vi "acq_eeg_read.vi"(7 "Marker Queue":refnum<queue>, 8 "error in (no error)":errorcluster, 10 "variant in":variant, 11 "eeg_device":T1) -> (0 "error out":errorcluster, 1 "Next Acq State":string, 2 "Variant out":variant, 3 "eeg samples":dbl[][](array[numeric]), 5 "Marker Queue Out":refnum<queue>)   [LabVIEW 2013]
uses:
  <vilib>/NIOSC/Address Space Node.ctl
  gui/type_def/device.ctl
  <vilib>/NI/Emotiv Toolkit/Emotiv Task.lvclass
  <vilib>/NI/Emotiv Toolkit/Utilities/EE DataChannels_enum.ctl
  <vilib>/OpenBCI/Comm Protocol/Control Def/openbci_device.ctl
  <vilib>/OpenBCI/Comm Protocol/Control Def/channel_count.ctl
  gui/type_def/file_stream.ctl
  <vilib>/NIOSC/Argument to Float32 Data.vi
  <vilib>/NIOSC/Generate Error.vi
  <vilib>/NIOSC/NI_OSC.lvlib
  <vilib>/NI/LabVIEW - NeuroSky Driver/NeuroSky Driver.lvlib
  <vilib>/NI/LabVIEW - NeuroSky Driver/NeuroSky Driver/ThinkGear Read/ThinkGear MultiSample Read Raw.vi
panel:
  out "Livesign Msg":bool
  out "ECG Chart":u32[](graph)
  out "Acc Chart":dbl[][](graph)
  out "Respiration Chart":u32[](graph)
  in  "NeuroSky Task Out":T2
  in  "muse cluster out":T4
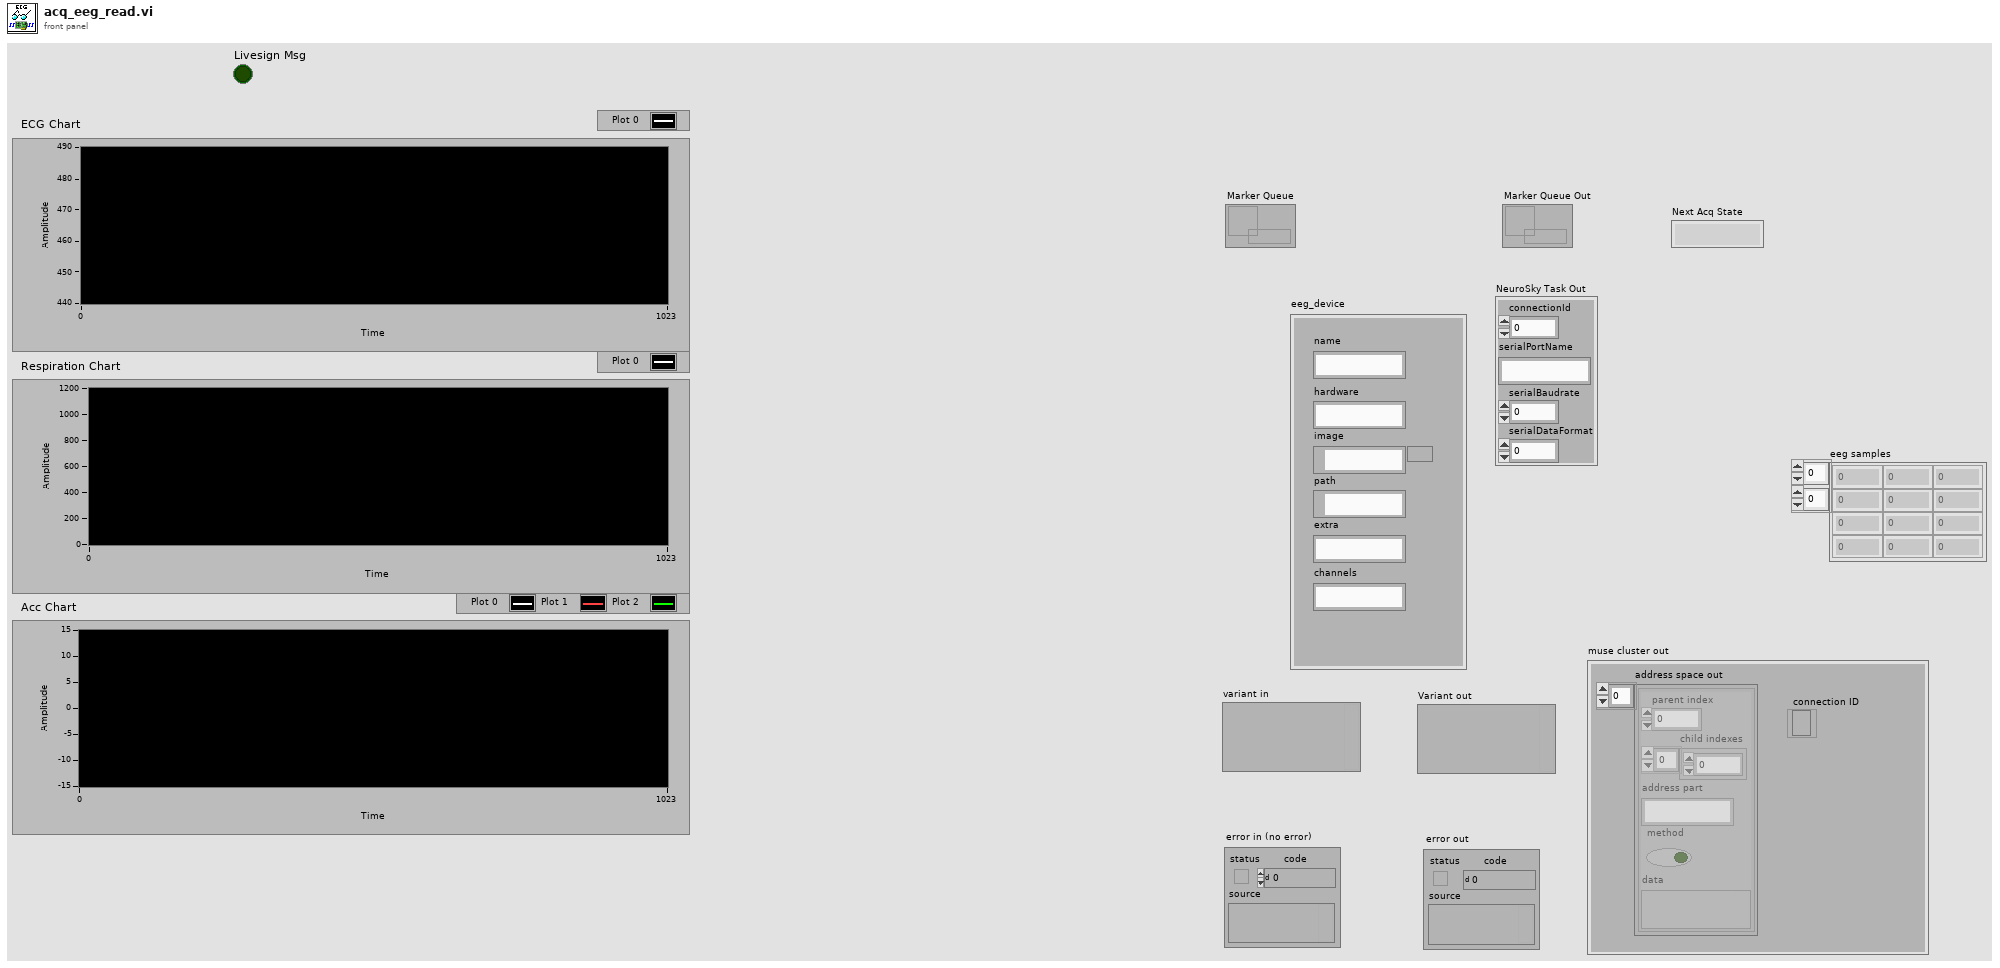
[diagram p1: front panel]
types:
  T1 = typedef "device.ctl" = cluster{"name":string, "hardware":string, "image":path, "path":path, "extra":string, "channels":string}
  T2 = cluster{"connectionId":i32, "serialPortName":string, "serialBaudrate":i32, "serialDataFormat":i32}
  T3 = typedef "NI_OSC.lvlib/Address Space Node.ctl" = cluster{"parent index":i32, "child indexes":i32[], "address part":string, "method":bool, "data":variant}
  T4 = cluster{"address space out":T3[], "connection ID":refnum<k5>}
  T5 = typedef "Emotiv Task.lvclass/EE DataChannels_enum.ctl" = enum8{"ED_COUNTER", "ED_INTERPOLATED", "ED_RAW_CQ", "ED_AF3", "ED_F7", "ED_F3", "ED_FC5", "ED_T7", "ED_P7", "ED_O1", "ED_O2", "ED_P8", "ED_T8", "ED_FC6", "ED_F4", "ED_F8", "ED_AF4", "ED_GYROX", "ED_GYROY", "ED_TIMESTAMP", "ED_ES_TIMESTAMP", "ED_FUNC_ID", "ED_FUNC_VALUE", "ED_MARKER", "ED_SYNC_SIGNAL"}
  T6 = typedef "openbci_device.ctl" = cluster{"COM port":refnum<visa-resource-name>, "n_ch (8)":T7, "delay_tx":u32}
  T7 = typedef "channel_count.ctl" = enum16{"8 Channels", "16 Channels"}
  T8 = typedef "file_stream.ctl" = cluster{"timestamp":timestamp, "data (2D array)":dbl[][], "Reading?":bool}
  T9 = typedef "NI_OSC.lvlib/Method Dispatching Info.ctl" = cluster{"method address":string, "message":string, "message timetag":u64, "data":variant}
  T10 = typedef "NI_OSC.lvlib/Argument.ctl" = cluster{"argument":string, "type tag":string}
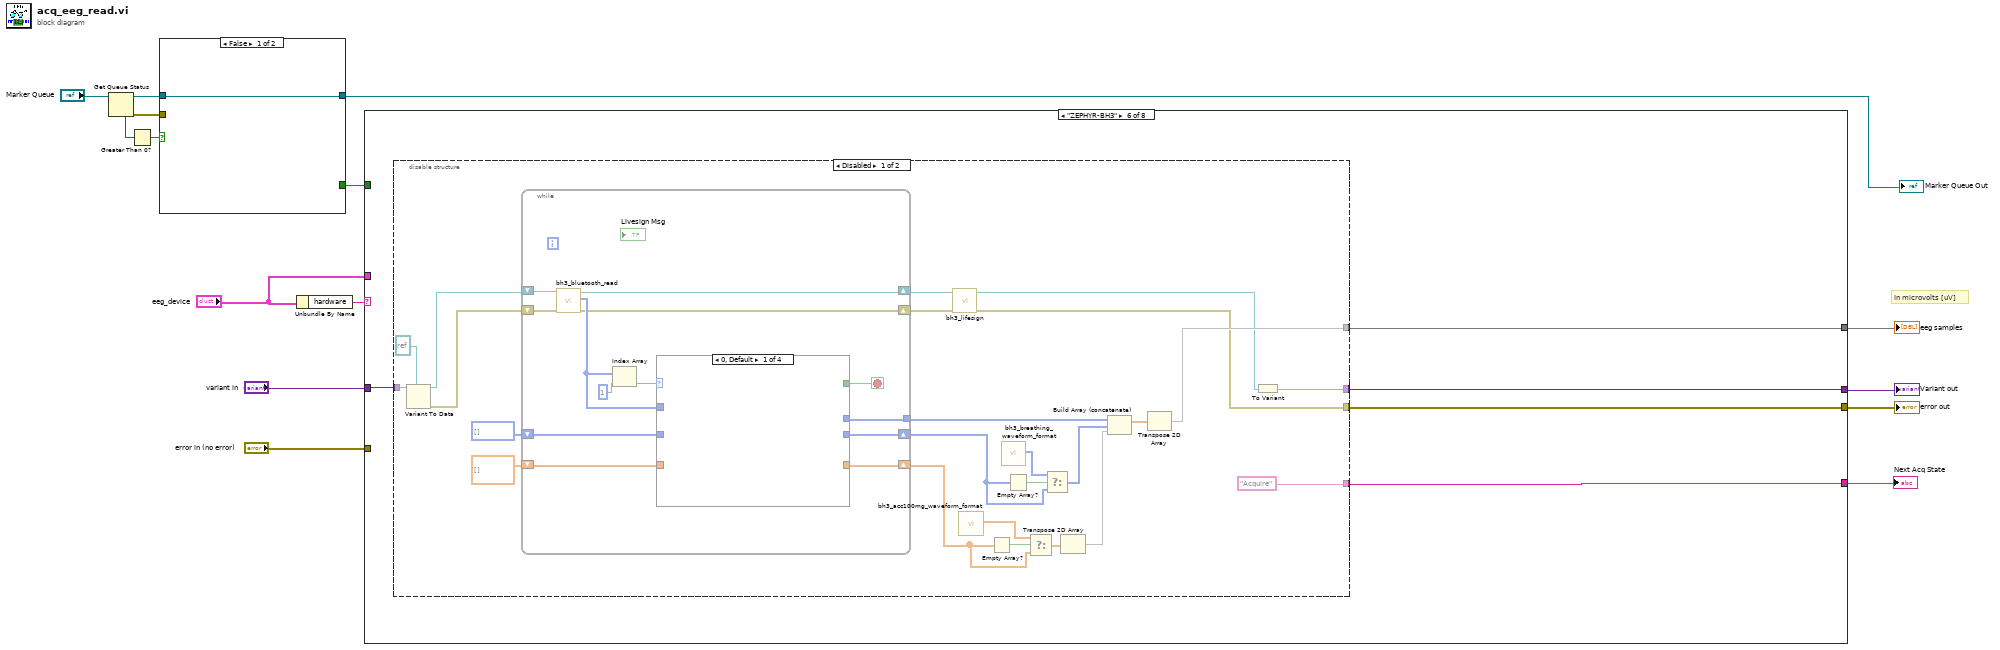
[diagram p0: block diagram]
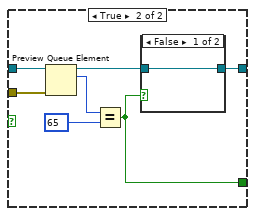
[diagram p2: hidden frame]
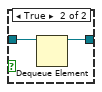
[diagram p3: hidden frame]
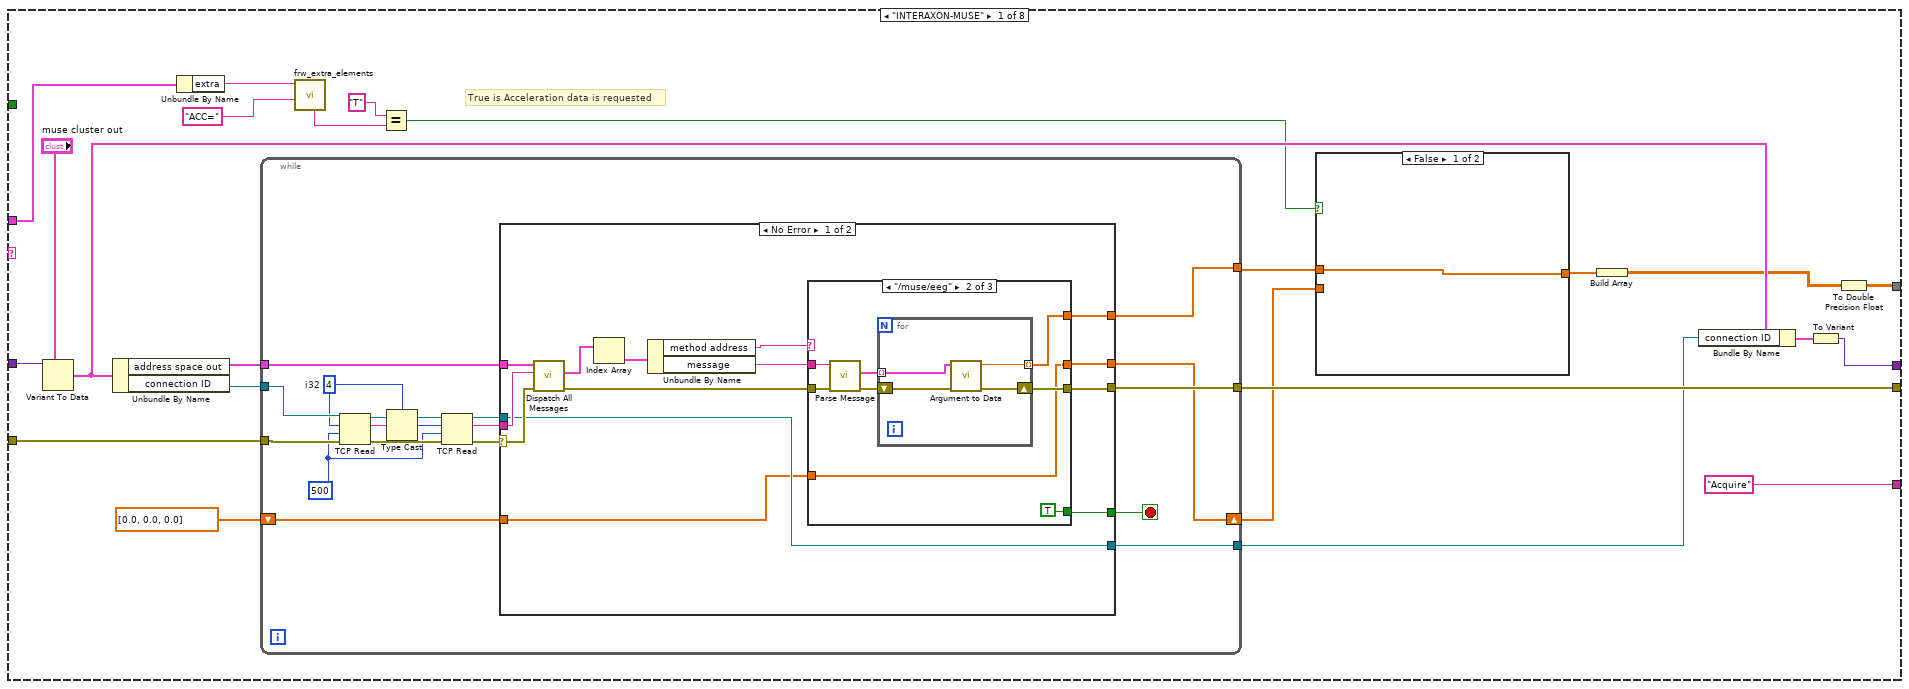
[diagram p4: hidden frame]
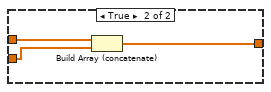
[diagram p5: hidden frame]
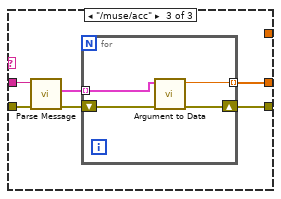
[diagram p7: hidden frame]
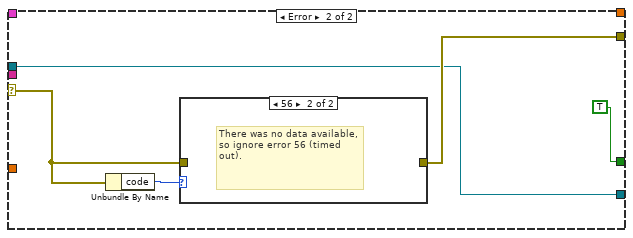
[diagram p8: hidden frame]
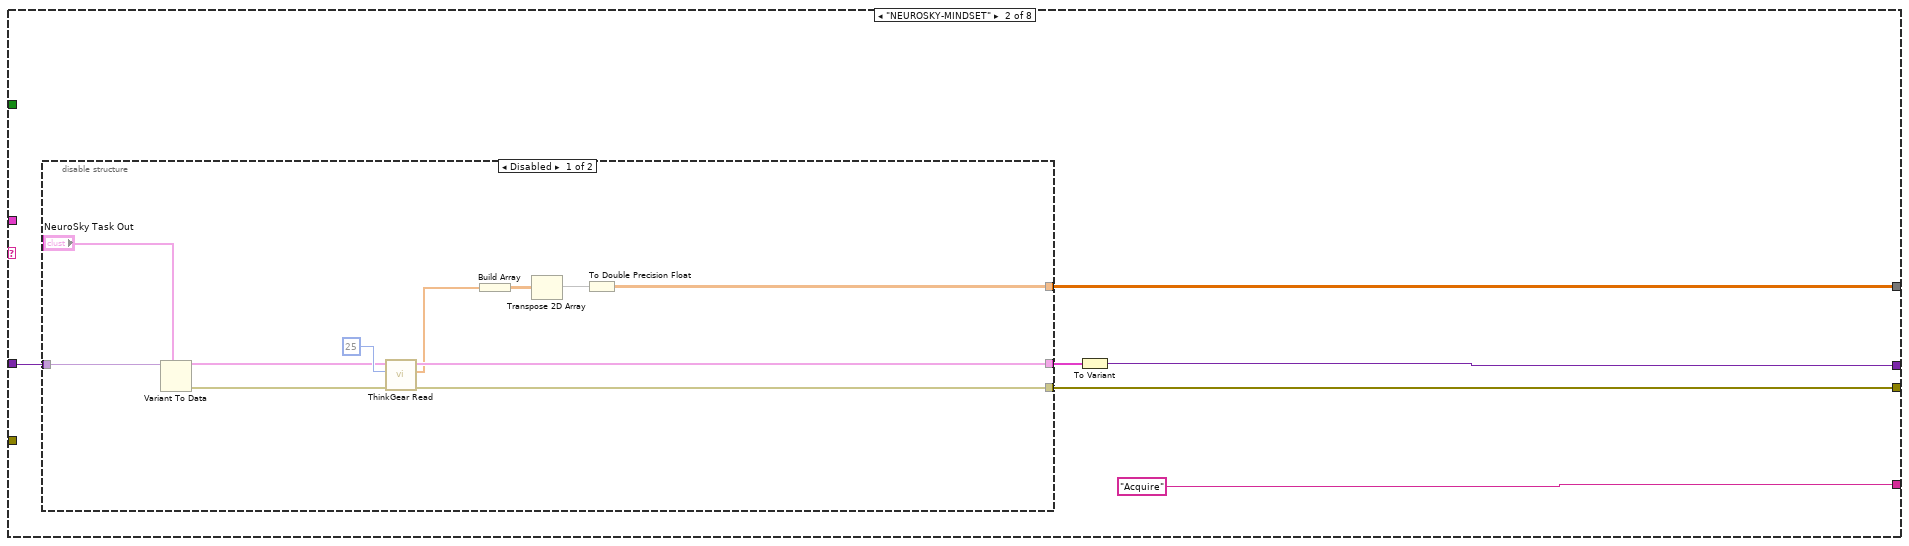
[diagram p10: hidden frame]
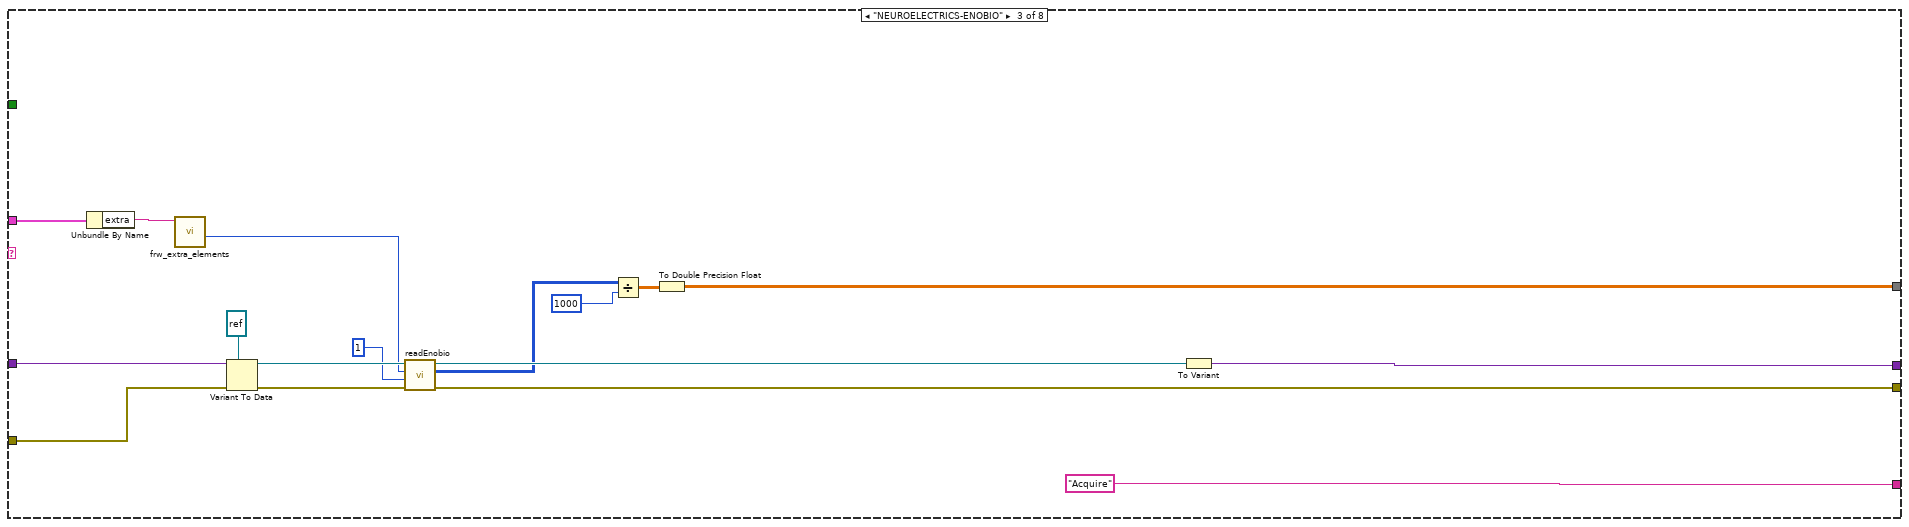
[diagram p12: hidden frame]
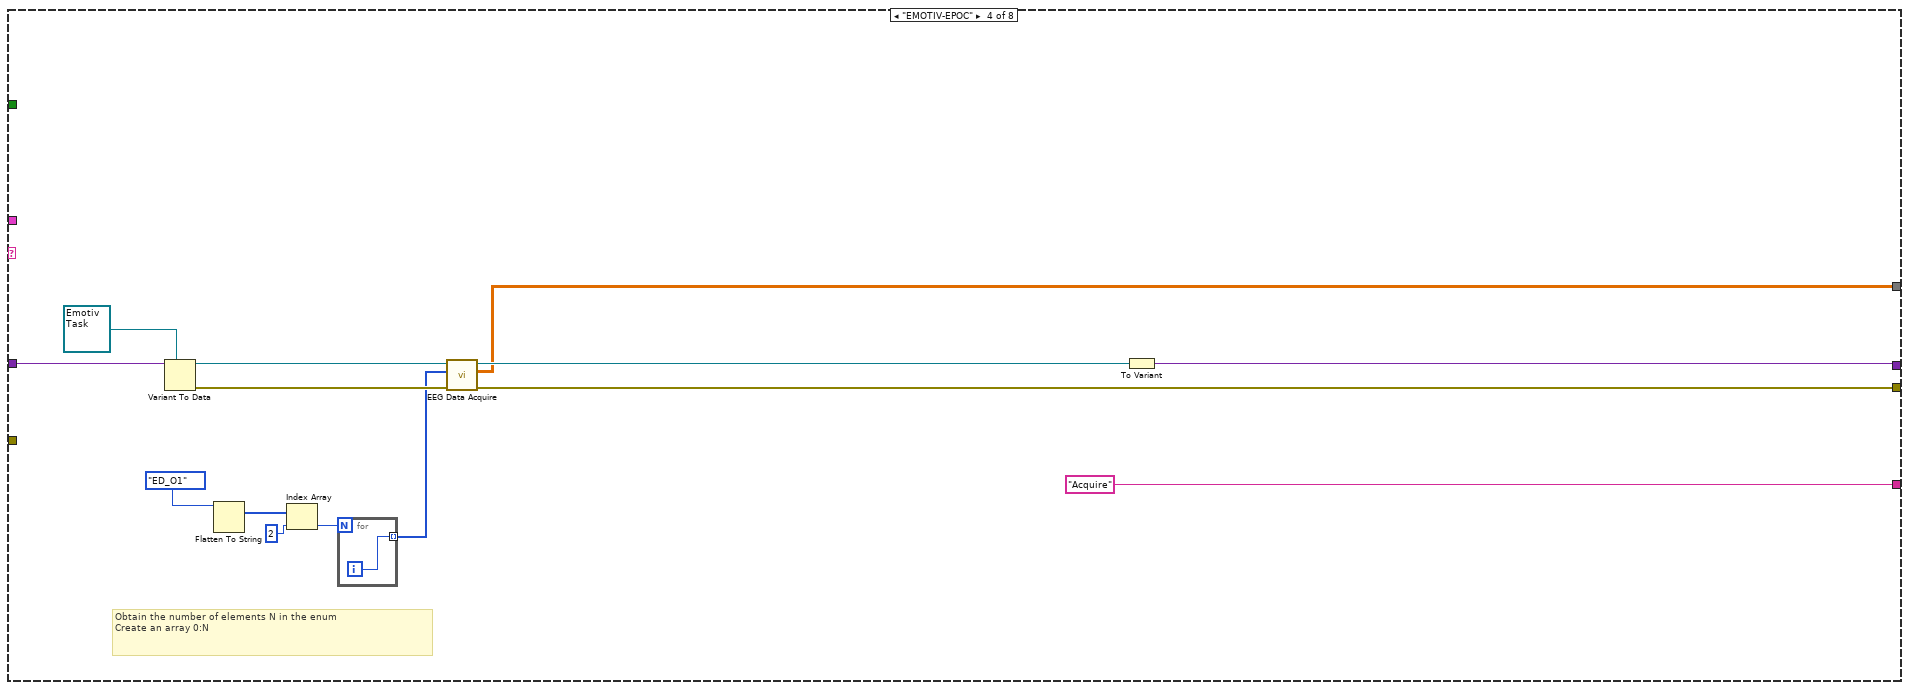
[diagram p13: hidden frame]
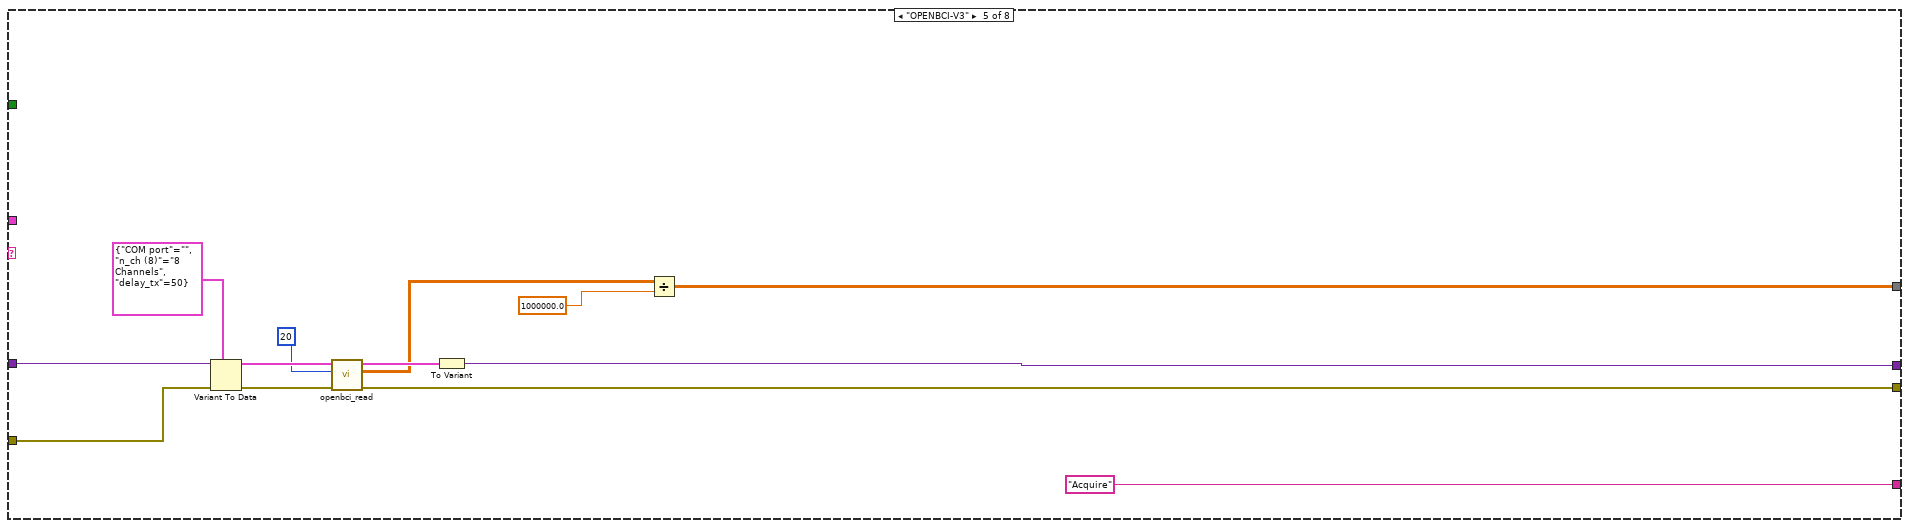
[diagram p14: hidden frame]
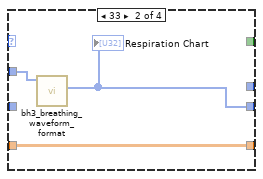
[diagram p15: hidden frame]
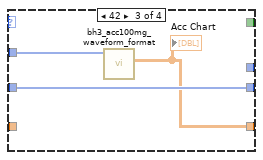
[diagram p16: hidden frame]
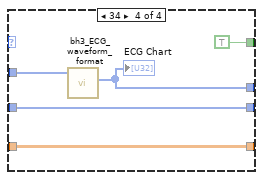
[diagram p17: hidden frame]
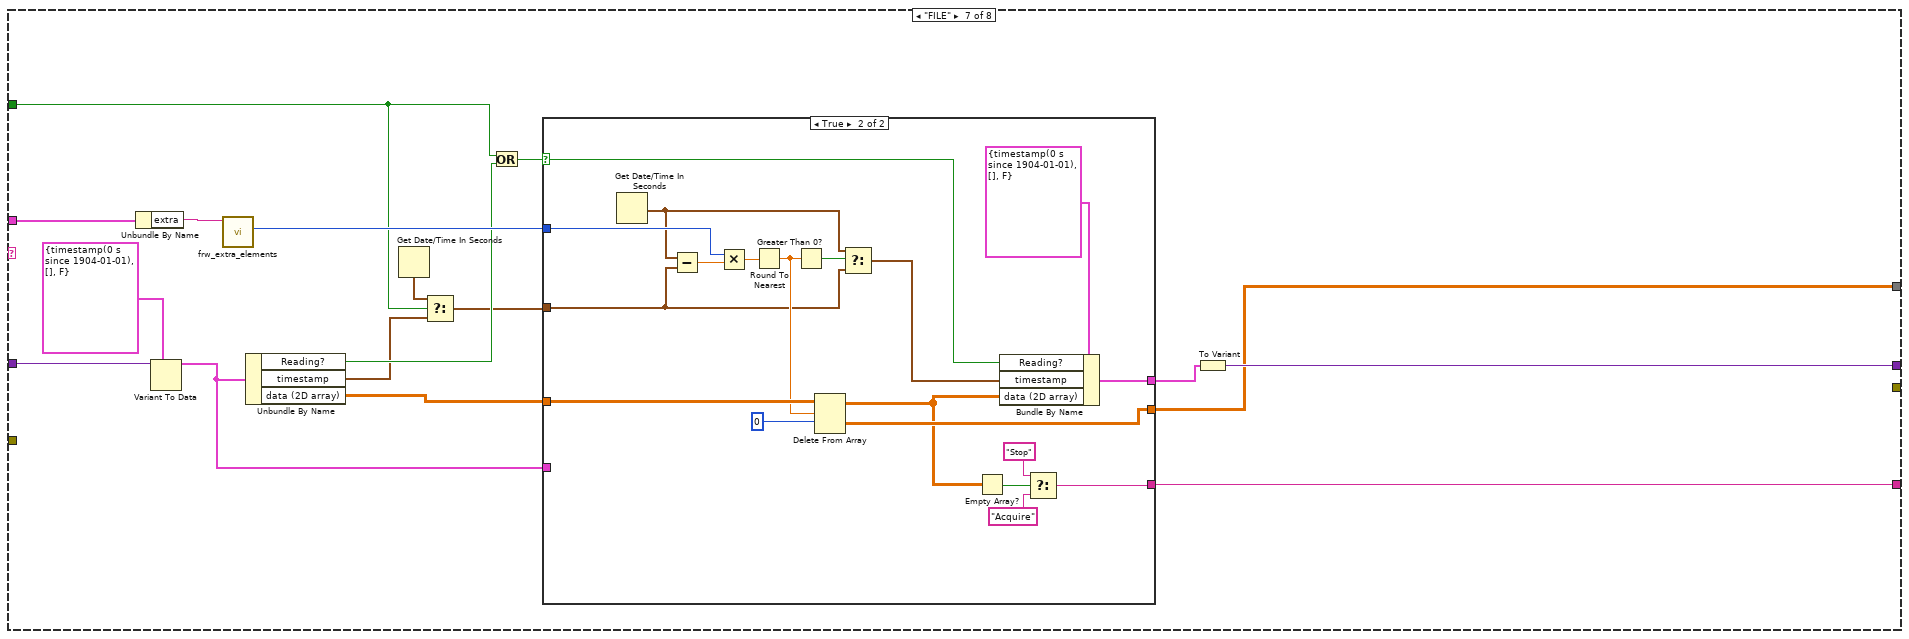
[diagram p19: hidden frame]
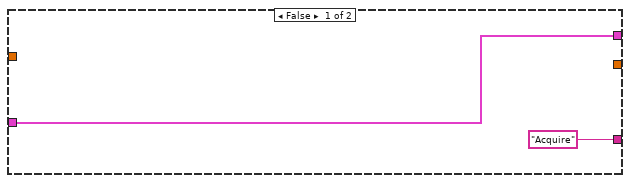
[diagram p20: hidden frame]
diagram:
  # "In microvolts [uV]"
  n1 = Get Queue Status(queue="Marker Queue") -> (queue out=w6:refnum<queue>, error out=w7:errorcluster, # elements in queue=w4:i32)  [unwired: 2 in, 5 out]
  n2 = Greater Than 0?(x=w4) -> (x > 0?=w5:bool)
  n3 = case shown="False" w5 {
    tunnel: w6 -> [w16 w23]
    tunnel: w7 -> [_ w22]
    tunnel: [w16 w19] -> w2
    tunnel: [_ w17] -> w1
    frame False {
    }
    frame True {
      n4 = Preview Queue Element(queue=w23, error in (no error)=w22) -> (queue out=w18:refnum<queue>, element=w21:u8)  [unwired: 1 in, 2 out]
      n5 = Equal?(x=w21, y=u8 65) -> (x = y?=w17:bool)
      n6 = case shown="False" w17 {
        tunnel: [w24 w26] -> w19
        tunnel: w18 -> [w24 w25]
        frame False {
        }
        frame True {
          n7 = Dequeue Element(queue=w25) -> (queue out=w26:refnum<queue>)  [unwired: 2 in, 3 out]
        }
      }
    }
  }
  "Marker Queue Out" <- w2
  n8 = Unbundle By Name("eeg_device") -> ("hardware"=w15:string)
  n9 = case shown="\"ZEPHYR-BH3\"" w15 {
    tunnel: "eeg_device" -> [w39 _ w135 _ _ _ w244 _]
    tunnel: "error in (no error)" -> [w46 _ w147 _ w173 _ _ w272]
    tunnel: [w45 w120 w141 w155 w169 w179 _ w272] -> w9
    tunnel: [w30 w117 w140 w151 w165 w180 w241 _] -> w13
    tunnel: "variant in" -> [w49 w121 w148 w152 w176 w182 w247 w271]
    tunnel: [w42 w119 w143 w154 w170 w181 w245 w271] -> w11
    tunnel: ["Acquire" ("Message") "Acquire" ("Message") "Acquire" ("Message") "Acquire" ("Message") "Acquire" ("Message") w178 w236 "Acquire" ("Message")] -> w8
    tunnel: w1 -> [_ _ _ _ _ _ w235 _]
    frame "INTERAXON-MUSE" {
      # "True is Acceleration data is requested"
      n10 = Variant To Data(type="muse cluster out", Variant=w49) -> (data=w41:T4)  [unwired: 1 in, 1 out]
      n11 = Unbundle By Name(w41) -> ("address space out"=w48:T3[], "connection ID"=w47:refnum<k5>)
      n12 = Unbundle By Name(w39) -> ("extra"=w38:string)
      n13 = while {
        tunnel: w48 -> [w71]
        tunnel: w47 -> [w70]
        tunnel: w46 -> [w61]
        tunnel: [w60] -> w45
        tunnel: [w59] -> w44
        tunnel: [w57] -> w32
        shift-right: [w55] -> w31
        shift-left: sgl[] [0.0, 0.0, 0.0] -> [w54]
        stop <- w56 stop-if-true
        w58 = 500 ("timeout ms (25000)")
        w62 = 4  # i32
        n14 = TCP Read(connection ID=w70, bytes to read=w62, error in (no error)=w61, 9:w58) -> (connection ID out=w67:refnum<k5>, data out=w63:string, error out=w69:errorcluster)  [unwired: 1 in]
        n15 = Type Cast(type=w62, x=w63) -> (*(type *) &x=w64:i32)
        n16 = TCP Read(connection ID=w67, bytes to read=w64, error in (no error)=w69, 9:w58) -> (connection ID out=w66:refnum<k5>, data out=w65:string, error out=w68:errorcluster)  [unwired: 1 in]
        n17 = case shown="No Error" w68 {
          selector: w68 -> [w84 w113]
          tunnel: w66 -> [w79 w111]
          tunnel: [w79 w111] -> w59
          tunnel: [w82 w112] -> w60
          tunnel: w65 -> [w81 _]
          tunnel: w71 -> [w85 _]
          tunnel: [w80 _] -> w57
          tunnel: [w74 _] -> w55
          tunnel: [w73 TRUE] -> w56
          tunnel: w54 -> [w72 _]
          frame No Error {
            n18 = call <vilib>:"Dispatch All Messages.vi"("error in"=w84, "packet"=w81, "address space in"=w85) -> ("error out"=w83:errorcluster, "method dispatching info"=w76:T9[])  [unwired: 6 in, 1 out]
            n19 = Index Array(array=w76) -> (element=w75:T9)  [unwired: 1 in]
            n20 = Unbundle By Name(w75) -> ("method address"=w78:string, "message"=w77:string)
            n21 = case shown="\"/muse/eeg\"" w78 {
              tunnel: w83 -> [w87 w95 w105]
              tunnel: [w87 w92 w101] -> w82
              tunnel: w77 -> [_ w94 w104]
              tunnel: [_ w90 _] -> w80
              tunnel: [w86 w88 w100] -> w74
              tunnel: [_ TRUE _] -> w73
              tunnel: w72 -> [w86 w88 _]
              frame Default {
              }
              frame "/muse/eeg" {
                n22 = call <vilib>:"Parse Message.vi"("error in"=w95, "message"=w94) -> ("error out"=w93:errorcluster, "arguments"=w91:T10[])  [unwired: 7 in, 1 out]
                n23 = for {
                  tunnel: w91 -> [w98] mode=indexing
                  tunnel: [w97] -> w90 mode=indexing
                  shift-right: [w96] -> w92
                  shift-left: w93 -> [w99]
                  n24 = call-poly <vilib>:"Argument to Data.vi"("error in"=w99, "float32 argument"=w98) -> ("error out"=w96:errorcluster, "float32 data"=w97:sgl)  [unwired: 8 in]
                }
              }
              frame "/muse/acc" {
                n25 = call <vilib>:"Parse Message.vi"("error in"=w105, "message"=w104) -> ("error out"=w103:errorcluster, "arguments"=w102:T10[])  [unwired: 7 in, 1 out]
                n26 = for {
                  tunnel: w102 -> [w108] mode=indexing
                  tunnel: [w107] -> w100 mode=indexing
                  shift-right: [w106] -> w101
                  shift-left: w103 -> [w109]
                  n27 = call-poly <vilib>:"Argument to Data.vi"("error in"=w109, "float32 argument"=w108) -> ("error out"=w106:errorcluster, "float32 data"=w107:sgl)  [unwired: 8 in]
                }
              }
            }
          }
          frame Error {
            n28 = Unbundle By Name(w113) -> ("code"=w114:i32)
            n29 = case shown="56" w114 {
              tunnel: w113 -> [w115 _]
              tunnel: [w115 _] -> w112
              frame Default {
              }
              frame 56 {
                # "There was no data available, so ignore error 56 (timed out)."
              }
            }
          }
        }
      }
      n30 = call "frw_extra_elements.vi"("single field"="ACC=", "string"=w38) -> ("single string"=w35:string)  [unwired: 5 in, 4 out]
      n31 = Equal?(x="T", y=w35) -> (x = y?=w33:bool)
      n32 = case shown="False" w33 {
        tunnel: [w50 w51] -> w29
        tunnel: w32 -> [w50 w53]
        tunnel: w31 -> [_ w52]
        frame False {
        }
        frame True {
          n33 = Build Array (concatenate)(w53, w52) -> (w51:sgl[])
        }
      }
      n34 = Build Array(w29) -> (w28:sgl[][])
      n35 = Bundle By Name(cluster=w41, "connection ID"=w44) -> (w43:T4)
      n36 = To Variant(anything=w43) -> (Variant=w42:variant)
      n37 = To Double Precision Float(number=w28) -> (double precision float=w30:dbl[][])
    }
    frame "NEUROSKY-MINDSET" {
      n38 = disable-structure shown="Disabled" {
        disable-tunnel: w121 -> [w132 _]
        disable-tunnel: [w127 _] -> w120
        disable-tunnel: [w126 _] -> w118
        disable-tunnel: [w122 _] -> w117
        frame Disabled {
          n39 = Variant To Data(type="NeuroSky Task Out", Variant=w132) -> (data=w128:T2, error out=w129:errorcluster)  [unwired: 1 in]
          n40 = call-poly <vilib>:"ThinkGear Read.vi"("error in (no error)"=w129, "Samples to Read"=25, "NeuroSky Task In"=w128) -> ("error out"=w127:errorcluster, "Data Out"=w125:sgl[], "NeuroSky Task Out"=w126:T2)  [unwired: 6 in]
          n41 = Build Array(w125) -> (w124:sgl[][])
          n42 = Transpose 2D Array(2D array=w124) -> (transposed array=w123:sgl[][])
          n43 = To Double Precision Float(number=w123) -> (double precision float=w122:dbl[][])
        }
        frame Enabled {
        }
      }
      n44 = To Variant(anything=w118) -> (Variant=w119:variant)
    }
    frame "NEUROELECTRICS-ENOBIO" {
      n45 = Unbundle By Name(w135) -> ("extra"=w134:string)
      n46 = call "frw_extra_elements.vi"("string"=w134) -> ("#ch"=w133:i32)  [unwired: 6 in, 4 out]
      n47 = Variant To Data(error in=w147, type=refnum<k5> refnum ("connection ID"), Variant=w148) -> (data=w146:refnum<k5>, error out=w145:errorcluster)
      n48 = call "readEnobio.vi"("error in (no error)"=w145, "nSamples"=1, "nChannels"=w133, "connection ID"=w146) -> ("error out"=w141:errorcluster, "output array"=w138:i32[][], "connection ID out"=w142:refnum<k5>)  [unwired: 5 in]
      n49 = Divide(x=w138, y=1000) -> (x/y=w139:dbl[][])
      n50 = To Double Precision Float(number=w139) -> (double precision float=w140:dbl[][])
      n51 = To Variant(anything=w142) -> (Variant=w143:variant)
    }
    frame "EMOTIV-EPOC" {
      # "Obtain the number of elements N in the enum\nCreate an array 0:N"
      n52 = Variant To Data(type=refnum<class "Emotiv Task.lvclass"> refnum ("Emotiv Task in"), Variant=w152) -> (data=w162:refnum<class "Emotiv Task.lvclass">, error out=w161:errorcluster)  [unwired: 1 in]
      n53 = Flatten To String(anything=EE_DataChannels_enum."ED_O1" ("EE_InputChannels_enum")) -> (type string=w158:i16[])  [unwired: 3 in, 2 out]
      n54 = Index Array(array=w158, index=2) -> (element=w157:i16)
      n55 = for {
        N: w157 -> [_]
        tunnel: [w164] -> w156 mode=indexing
        i -> [w164]
      }
      n56 = call <vilib>:"EEG Data Acquire.vi"("error in (no error)"=w161, "channel_array"=w156, "Emotiv Task in"=w162) -> ("error out"=w155:errorcluster, "EEG data"=w151:dbl[][], "Emotiv Task out"=w153:refnum<class "Emotiv Task.lvclass">)  [unwired: 5 in, 1 out]
      n57 = To Variant(anything=w153) -> (Variant=w154:variant)
    }
    frame "OPENBCI-V3" {
      n58 = Variant To Data(error in=w173, type=T6 {"COM port"="", "n_ch (8)"=enum."8 Channels", "delay_tx"=50} ("OBCI dev in"), Variant=w176) -> (data=w175:T6, error out=w174:errorcluster)
      n59 = call <vilib>:"openbci_read.vi"("error in"=w174, "N samples (2)"=20, "OBCI dev in"=w175) -> ("error out"=w169:errorcluster, "EEG data"=w167:dbl[][], "OBCI dev out"=w171:T6)  [unwired: 5 in, 1 out]
      n60 = To Variant(anything=w171) -> (Variant=w170:variant)
      n61 = Divide(x=w167, y=1000000.0) -> (x/y=w165:dbl[][])
    }
    frame "ZEPHYR-BH3" {
      n62 = disable-structure shown="Disabled" {
        disable-tunnel: w182 -> [w192 _]
        disable-tunnel: [w189 _] -> w181
        disable-tunnel: [w188 _] -> w180
        disable-tunnel: [w184 _] -> w179
        disable-tunnel: ["Acquire" ("Message") _] -> w178
        frame Disabled {
          n63 = Variant To Data(type=refnum<k31> refnum ("bt connection ID out"), Variant=w192) -> (data=w191:refnum<k31>, error out=w190:errorcluster)  [unwired: 1 in]
          n64 = while {
            shift-right: [w211] -> w186
            shift-left: w191 -> [w214]
            shift-right: [w212] -> w187
            shift-left: w190 -> [w213]
            tunnel: [w215] -> w194
            shift-right: [w210] -> w198
            shift-left: u32[] [] ("breathing data") -> [w209]
            shift-right: [w208] -> w202
            shift-left: dbl[][] [] ("acc (G)") -> [w207]
            stop <- w216 stop-if-true
            n65 = call <vilib>:"bh3_bluetooth_read.vi"("error in (no error)"=w213, "bt connection ID in"=w214) -> ("error out"=w212:errorcluster, "response byte array"=w217:u8[], "bt connection ID out"=w211:refnum<k31>)  [unwired: 7 in]
            n66 = Index Array(array=w217, index=1) -> (element=w219:u8)
            n67 = case shown="0, Default" w219 {
              tunnel: w217 -> [_ w222 w225 w230]
              tunnel: [_ _ _ TRUE] -> w216
              tunnel: [_ _ _ w228] -> w215
              tunnel: [_ w221 w224 w227] -> w210
              tunnel: w209 -> [_ _ w224 w227]
              tunnel: [_ w220 w223 w226] -> w208
              tunnel: w207 -> [_ w220 _ w226]
              frame 0, Default {
              }
              frame 33 {
                n68 = call <vilib>:"bh3_breathing_waveform_format.vi"("Breathing Waveform Packet"=w222) -> ("breathing data"=w221:u32[])  [unwired: 5 in, 5 out]
                "Respiration Chart" <- w221
              }
              frame 42 {
                n69 = call <vilib>:"bh3_acc100mg_waveform_format.vi"("Acc 100mg Waveform Packet"=w225) -> ("acc (G)"=w223:dbl[][])  [unwired: 5 in, 5 out]
                "Acc Chart" <- w223
              }
              frame 34 {
                n70 = call <vilib>:"bh3_ECG_waveform_format.vi"("ECG Waveform Packet"=w230) -> ("ECG data"=w228:u32[])  [unwired: 5 in, 5 out]
                "ECG Chart" <- w228
              }
            }
          }
          n71 = call <vilib>:"bh3_lifesign.vi"("error in (no error)"=w187, "bt connection ID in"=w186) -> ("error out"=w184:errorcluster, "bt connection ID out"=w185:refnum<k31>)  [unwired: 8 in]
          n72 = call <vilib>:"bh3_acc100mg_waveform_format.vi"() -> ("acc (G)"=w203:dbl[][])  [unwired: 6 in, 5 out]
          n73 = Empty Array?(array=w202) -> (empty?=w201:bool)
          n74 = call <vilib>:"bh3_breathing_waveform_format.vi"() -> ("breathing data"=w196:u32[])  [unwired: 6 in, 5 out]
          n75 = Empty Array?(array=w198) -> (empty?=w197:bool)
          n76 = Select(t=w203, s=w201, f=w202) -> (s? t:f=w205:dbl[][])
          n77 = Select(t=w196, s=w197, f=w198) -> (s? t:f=w199:u32[])
          n78 = Transpose 2D Array(2D array=w205) -> (transposed array=w206:dbl[][])
          n79 = Build Array (concatenate)(w194, w199, w206) -> (w195:dbl[][])
          n80 = Transpose 2D Array(2D array=w195) -> (transposed array=w188:dbl[][])
          n81 = To Variant(anything=w185) -> (Variant=w189:variant)
        }
        frame Enabled {
        }
      }
    }
    frame "FILE" {
      n82 = Unbundle By Name(w244) -> ("extra"=w243:string)
      n83 = Variant To Data(type=T8 {"timestamp"=timestamp(0 s since 1904-01-01), "data (2D array)"=[], "Reading?"=FALSE} ("output cluster"), Variant=w247) -> (data=w231:T8)  [unwired: 1 in, 1 out]
      n84 = call "frw_extra_elements.vi"("string"=w243) -> ("fs"=w242:i32)  [unwired: 6 in, 4 out]
      n85 = Unbundle By Name(w231) -> ("Reading?"=w237:bool, "timestamp"=w234:timestamp, "data (2D array)"=w239:dbl[][])
      n86 = Get Date/Time In Seconds() -> (seconds since 1Jan1904=w232:timestamp)
      n87 = Select(t=w232, s=w235, f=w234) -> (s? t:f=w233:timestamp)
      n88 = Or(x=w235, y=w237) -> (x .or. y?=w238:bool)
      n89 = case shown="True" w238 {
        selector: w238 -> [_ w261]
        tunnel: w242 -> [_ w267]
        tunnel: [_ w265] -> w241
        tunnel: [w248 w263] -> w240
        tunnel: w239 -> [_ w262]
        tunnel: ["Acquire" ("Message") w255] -> w236
        tunnel: w233 -> [_ w250]
        tunnel: w231 -> [w248 _]
        frame False {
        }
        frame True {
          n90 = Get Date/Time In Seconds() -> (seconds since 1Jan1904=w253:timestamp)
          n91 = Subtract(x=w253, y=w250) -> (x-y=w268:dbl)
          n92 = Multiply(x=w267, y=w268) -> (x*y=w266:dbl)
          n93 = Round To Nearest(number=w266) -> (nearest integer value=w251:dbl)
          n94 = Greater Than 0?(x=w251) -> (x > 0?=w254:bool)
          n95 = Delete From Array(array=w262, length=w251, index (row)=0) -> (deleted portion=w265:dbl[][], array with subset deleted=w259:dbl[][])  [unwired: 1 in]
          n96 = Select(t=w253, s=w254, f=w250) -> (s? t:f=w252:timestamp)
          n97 = Empty Array?(array=w259) -> (empty?=w257:bool)
          n98 = Bundle By Name(cluster=T8 {"timestamp"=timestamp(0 s since 1904-01-01), "data (2D array)"=[], "Reading?"=FALSE} ("output cluster"), "Reading?"=w261, "timestamp"=w252, "data (2D array)"=w259) -> (w263:T8)
          n99 = Select(t="Stop" ("Message"), s=w257, f="Acquire" ("Message")) -> (s? t:f=w255:string)
        }
      }
      n100 = To Variant(anything=w240) -> (Variant=w245:variant)
    }
    frame Default {
      n101 = One Button Dialog(message="How did you get here?") -> ()  [unwired: 1 in, 1 out]
    }
  }
  "error out" <- w9
  "eeg samples" <- w13
  "Variant out" <- w11
  "Next Acq State" <- w8
